vi "Fault_Table_Read.vi"(2 "ERD Data Out":T2[](array[typedef]) {"ERD Number" format="%.0x"}, 5 "Error In":errorcluster) -> (11 "Fault Table 0":T1, 13 "Fault Table 1":T1, 16 "Fault Table 2":T1, 17 "Fault Table 3":T1, 18 "Fault Table 4":T1, 19 "Error Out":errorcluster)   [LabVIEW 2014]
uses:
  Utility/Labview GEA2 Toolkit v2.1/type defs/ERD Read Data Out.ctl
  type defs/Fault_Table_Info.ctl
  Utility/Labview GEA2 Toolkit v2.1/library/GEA2_Toolkit.lvlib
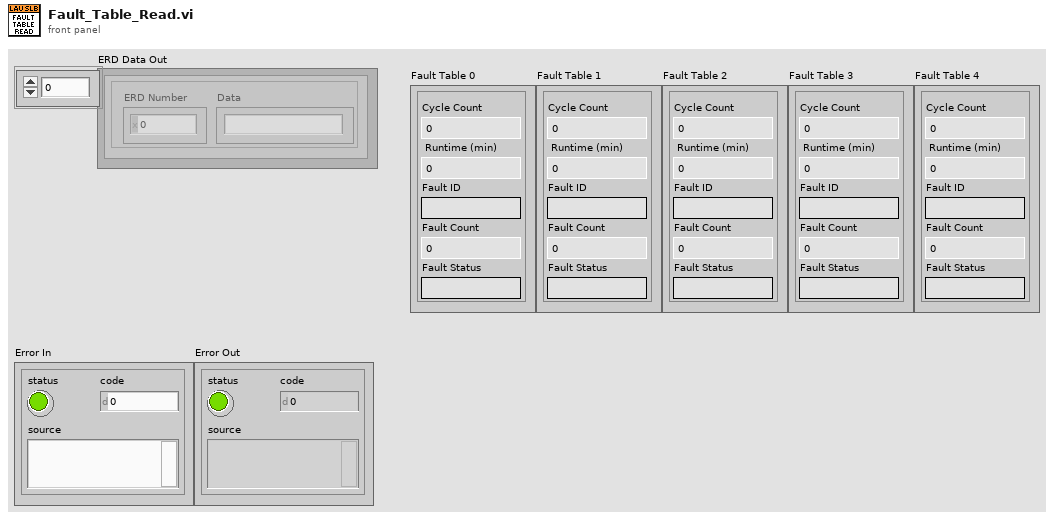
[diagram p1: front panel]
types:
  T1 = typedef "Fault_Table_Info.ctl" = cluster{"Cycle Count":u32, " Runtime (min) ":u32, "Fault Status":string, "Fault ID":string, "Fault Count":u16}
  T2 = typedef "GEA2_Toolkit.lvlib/ERD Read Data Out.ctl" = cluster{"ERD Number":u16, "Data":string}
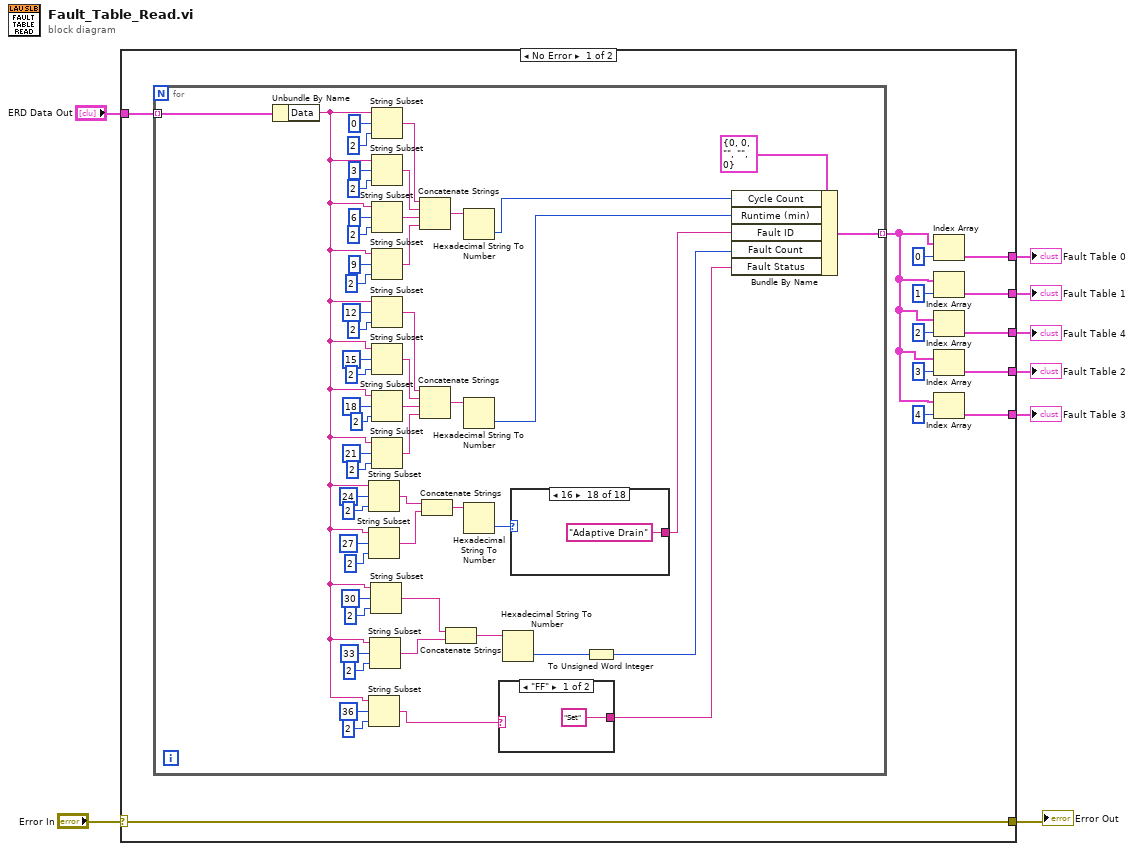
[diagram p0: block diagram]
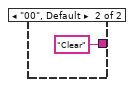
[diagram p2: hidden frame]
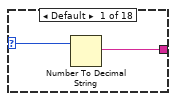
[diagram p3: hidden frame]
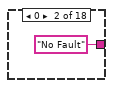
[diagram p4: hidden frame]
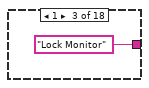
[diagram p5: hidden frame]
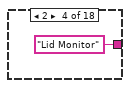
[diagram p6: hidden frame]
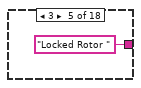
[diagram p7: hidden frame]
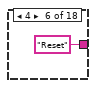
[diagram p8: hidden frame]
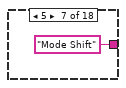
[diagram p9: hidden frame]
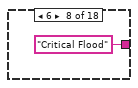
[diagram p10: hidden frame]
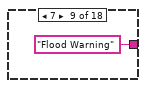
[diagram p11: hidden frame]
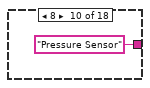
[diagram p12: hidden frame]
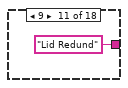
[diagram p13: hidden frame]
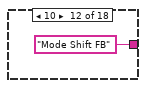
[diagram p14: hidden frame]
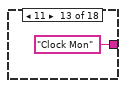
[diagram p15: hidden frame]
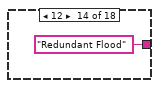
[diagram p16: hidden frame]
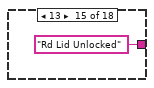
[diagram p17: hidden frame]
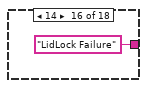
[diagram p18: hidden frame]
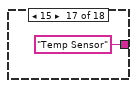
[diagram p19: hidden frame]
diagram:
  n1 = case shown="No Error" "Error In" {
    selector: "Error In" -> [w20 w97]
    tunnel: [w20 w97] -> w7
    tunnel: "ERD Data Out" -> [w21 _]
    tunnel: [w14 _] -> w5
    tunnel: [w13 _] -> w4
    tunnel: [w12 _] -> w3
    tunnel: [w11 _] -> w2
    tunnel: [w10 _] -> w1
    frame No Error {
      n2 = for {
        tunnel: w21 -> [w75] mode=indexing
        tunnel: [w24] -> w9 mode=indexing
        n3 = Unbundle By Name(w75) -> ("Data"=w32:string)
        n4 = String Subset(string=w32, offset (0)=24, length (rest)=2 ("length (rest)")) -> (substring=w53:string)
        n5 = String Subset(string=w32, offset (0)=27, length (rest)=2 ("length (rest)")) -> (substring=w52:string)
        n6 = String Subset(string=w32, offset (0)=36, length (rest)=2 ("length (rest)")) -> (substring=w27:string)
        n7 = String Subset(string=w32, offset (0)=33, length (rest)=2 ("length (rest)")) -> (substring=w29:string)
        n8 = String Subset(string=w32, offset (0)=30, length (rest)=2 ("length (rest)")) -> (substring=w30:string)
        n9 = String Subset(string=w32, offset (0)=0, length (rest)=2 ("length (rest)")) -> (substring=w69:string)
        n10 = String Subset(string=w32, offset (0)=3, length (rest)=2 ("length (rest)")) -> (substring=w68:string)
        n11 = String Subset(string=w32, offset (0)=6, length (rest)=2 ("length (rest)")) -> (substring=w67:string)
        n12 = String Subset(string=w32, offset (0)=9, length (rest)=2 ("length (rest)")) -> (substring=w66:string)
        n13 = String Subset(string=w32, offset (0)=12, length (rest)=2 ("length (rest)")) -> (substring=w60:string)
        n14 = String Subset(string=w32, offset (0)=15, length (rest)=2 ("length (rest)")) -> (substring=w61:string)
        n15 = String Subset(string=w32, offset (0)=18, length (rest)=2 ("length (rest)")) -> (substring=w62:string)
        n16 = String Subset(string=w32, offset (0)=21, length (rest)=2 ("length (rest)")) -> (substring=w63:string)
        n17 = Concatenate Strings(w69, w68, w67, w66) -> (w65:string)
        n18 = Concatenate Strings(w60, w61, w62, w63) -> (w64:string)
        n19 = Concatenate Strings(w53, w52) -> (w51:string)
        n20 = Concatenate Strings(w30, w29) -> (w31:string)
        n21 = Hexadecimal String To Number(string=w65) -> (number=w23:u32)  [unwired: 2 in, 1 out]
        n22 = Hexadecimal String To Number(string=w64) -> (number=w38:u32)  [unwired: 2 in, 1 out]
        n23 = Hexadecimal String To Number(string=w51) -> (number=w22:u32)  [unwired: 2 in, 1 out]
        n24 = case shown="\"FF\"" w27 {
          tunnel: ["Set" "Clear"] -> w26
          frame "FF" {
          }
          frame "00", Default {
          }
        }
        n25 = Hexadecimal String To Number(string=w31) -> (number=w28:u32)  [unwired: 2 in, 1 out]
        n26 = case shown="16" w22 {
          selector: w22 -> [w79 _ _ _ _ _ _ _ _ _ _ _ _ _ _ _ _ _]
          tunnel: [w78 "No Fault" "Lock Monitor" "Lid Monitor" "Locked Rotor " "Reset" "Mode Shift" "Critical Flood" "Flood Warning" "Pressure Sensor" "Lid Redund" "Mode Shift FB" "Clock Mon" "Redundant Flood" "Rd Lid Unlocked" "LidLock Failure" "Temp Sensor" "Adaptive Drain"] -> w37
          frame Default {
            n27 = Number To Decimal String(number=w79) -> (decimal integer string=w78:string)  [unwired: 1 in]
          }
          frame 0 {
          }
          frame 1 {
          }
          frame 2 {
          }
          frame 3 {
          }
          frame 4 {
          }
          frame 5 {
          }
          frame 6 {
          }
          frame 7 {
          }
          frame 8 {
          }
          frame 9 {
          }
          frame 10 {
          }
          frame 11 {
          }
          frame 12 {
          }
          frame 13 {
          }
          frame 14 {
          }
          frame 15 {
          }
          frame 16 {
          }
        }
        n28 = To Unsigned Word Integer(number=w28) -> (unsigned 16bit integer=w25:u16)
        n29 = Bundle By Name(cluster=T1 {"Cycle Count"=0, " Runtime (min) "=0, "Fault Status"="", "Fault ID"="", "Fault Count"=0} ("Fault Table 0"), "Cycle Count"=w23, "Runtime (min)"=w38, "Fault ID"=w37, "Fault Count"=w25, "Fault Status"=w26) -> (w24:T1)
      }
      n30 = Index Array(array=w9, index=0) -> (element=w14:T1)
      n31 = Index Array(array=w9, index=1) -> (element=w13:T1)
      n32 = Index Array(array=w9, index=2) -> (element=w12:T1)
      n33 = Index Array(array=w9, index=3) -> (element=w11:T1)
      n34 = Index Array(array=w9, index=4) -> (element=w10:T1)
    }
    frame Error {
    }
  }
  "Error Out" <- w7
  "Fault Table 0" <- w5
  "Fault Table 1" <- w4
  "Fault Table 2" <- w2
  "Fault Table 3" <- w1
  "Fault Table 4" <- w3
